vi "SDCP FTOR.vi"(2 "error in (no error)":errorcluster, 3 "FID":u8[](array[numeric])) -> (0 "error out":errorcluster, 1 "Received frames":u8[][](array[numeric]))   [LabVIEW 2020]
uses:
  Typedefs/SDCP - Serial Port Control - Commands.ctl
  Typedefs/SDCP FTOR params.ctl
  <vilib>/Instr/_visa.llb/VISA Flush IO Buffer Mask.ctl
panel:
  out "Timeout errors\nframes":errorcluster[](array[cluster])
  out "timeout\nerrors\nACK":errorcluster[](array[cluster])
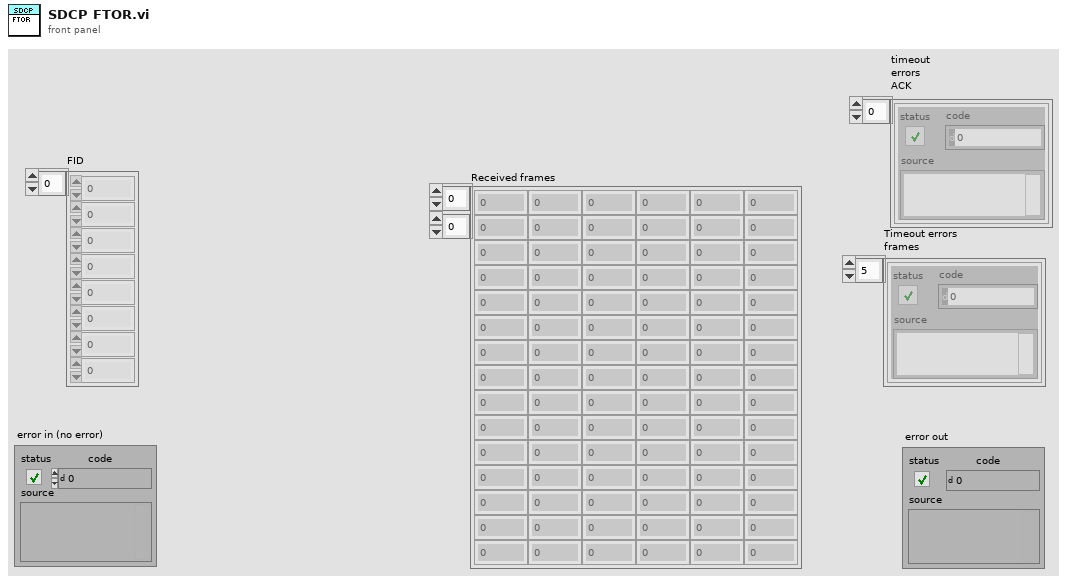
[diagram p1: front panel]
types:
  T1 = typedef "SDCP - Serial Port Control - Commands.ctl" = enum16{"Open", "Read", "Write", "Get instance", "Close"}
  T2 = typedef "SDCP FTOR params.ctl" = cluster{"FID_0":i32, "FID_1":i32, "FID_2":i32, "FID_3":i32, "FID_4":i32, "FID_5":i32, "FID_6":i32, "N_FIDs":i32, "REQ":bool, "ACK":bool}
  T3 = typedef "VISA Flush IO Buffer Mask.ctl" = u16
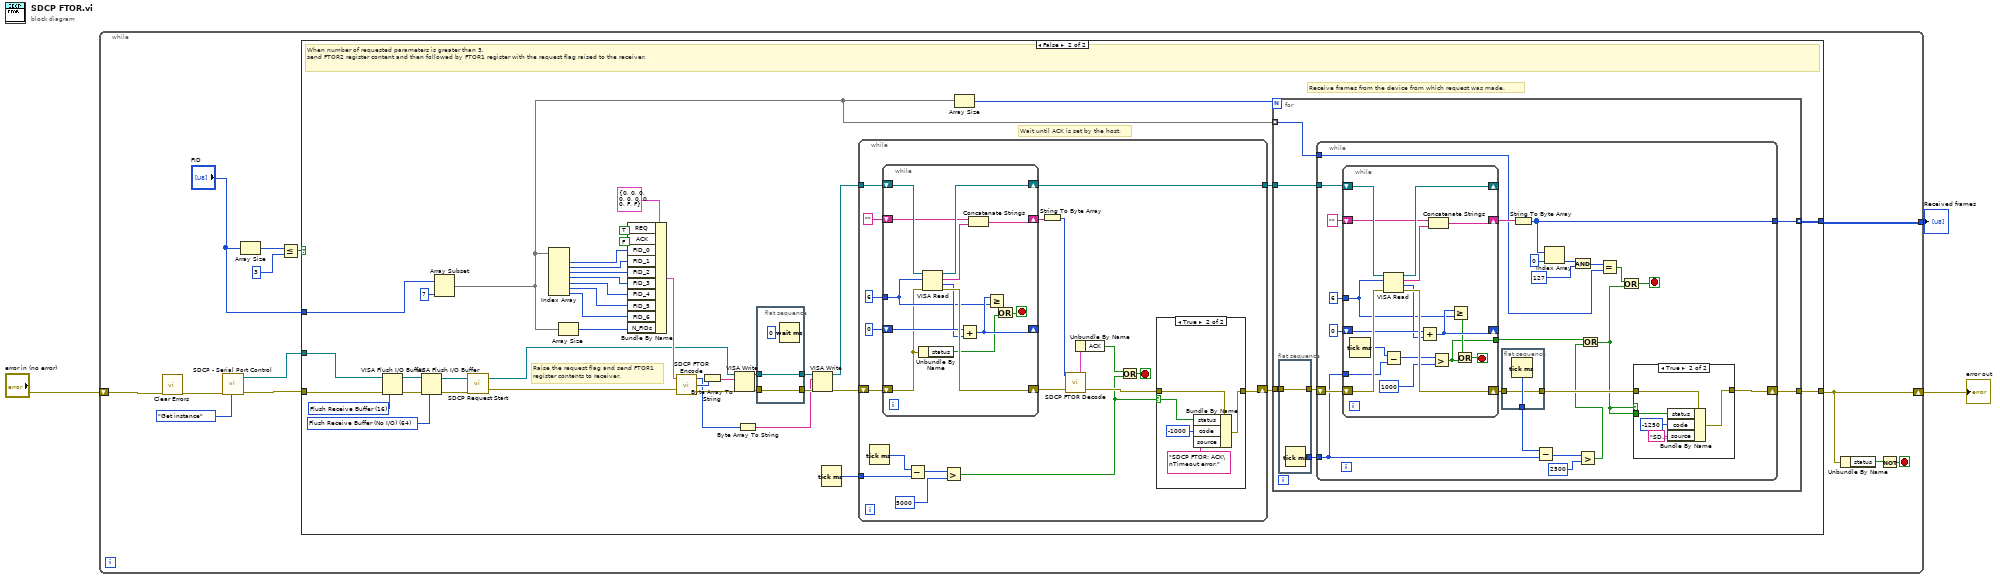
[diagram p0: block diagram]
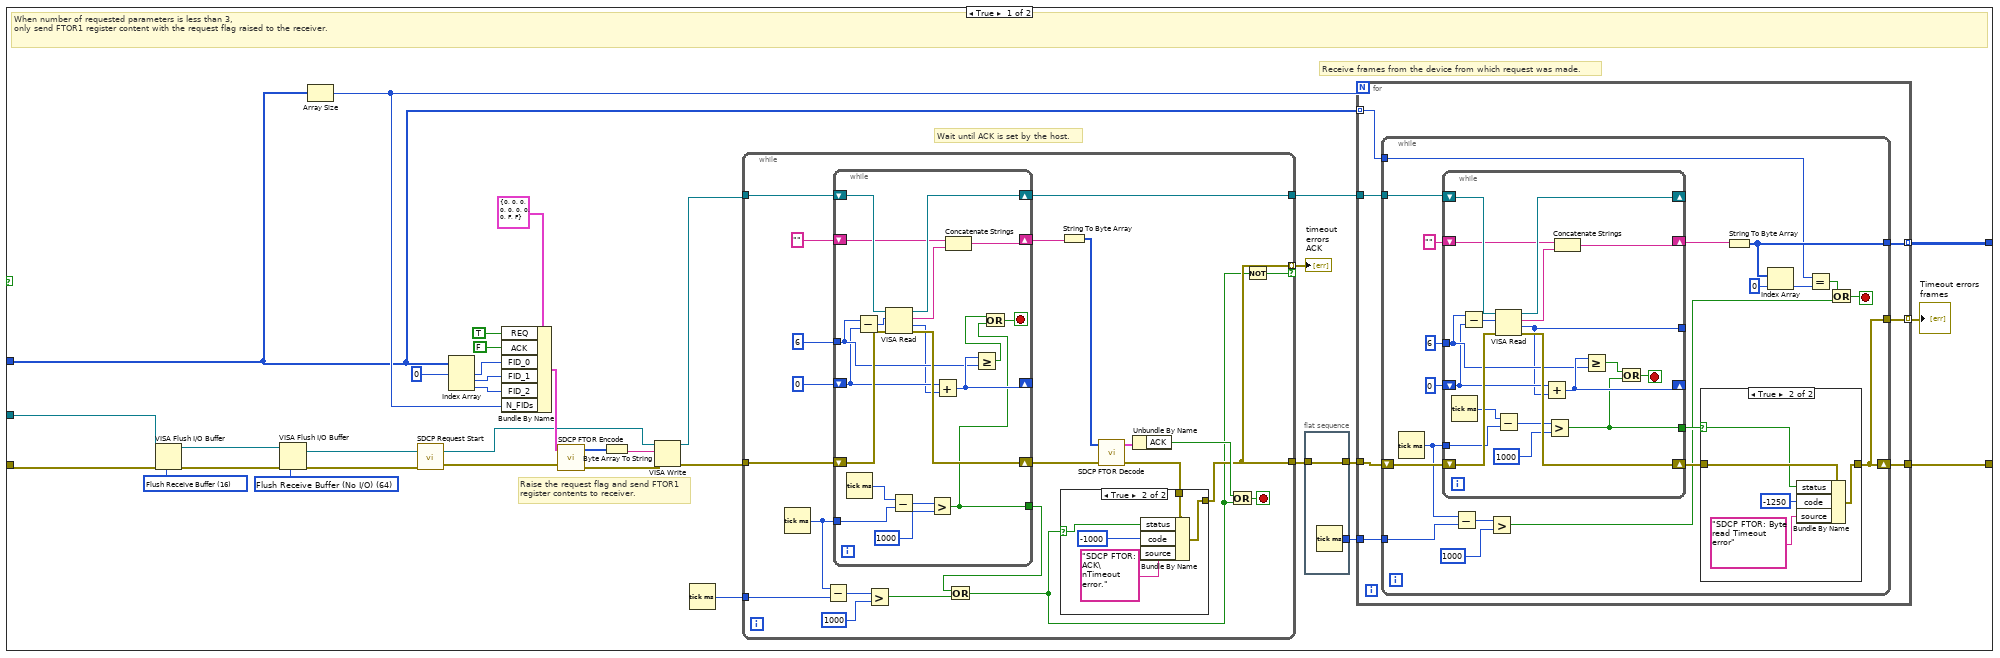
[diagram p2: hidden frame]
diagram:
  n1 = while {
    tunnel: [w9] -> w2
    shift-right: [w6] -> w3
    shift-left: "error in (no error)" -> [w8]
    stop <- w5 stop-if-true
    n2 = call <vilib>:"Clear Errors.vi"("error in (no error)"=w8) -> ("error out"=w7:errorcluster)  [unwired: 5 in, 1 out]
    n3 = call "SDCP - Serial Port Control.vi"("Command"=SDCP_-_Serial_Port_Control_-_Commands."Get instance", "error in (no error)"=w7) -> ("error out"=w12:errorcluster, "VISA out"=w10:refnum<visa-resource-name>)  [unwired: 6 in, 2 out]
    n4 = Array Size(array="FID") -> (size(s)=w15:i32)
    n5 = Less Or Equal?(x=w15, y=3) -> (x <= y?=w13:bool)
    n6 = case shown="False" w13 {
      tunnel: w12 -> [w32 w169]
      tunnel: "FID" -> [w33 w160]
      tunnel: w10 -> [w28 w164]
      tunnel: [w37 w182] -> w9
      tunnel: [w36 w181] -> w6
      frame True {
        w30 = T3 64 items=["Flush Receive Buffer"=16, "Write Transmit Buffer to Device"=32, "Flush Receive Buffer (No I/O)"=64, "Flush Transmit Buffer"=128] ("Mask")
        w31 = T3 16 items=["Flush Receive Buffer"=16, "Write Transmit Buffer to Device"=32, "Flush Receive Buffer (No I/O)"=64, "Flush Transmit Buffer"=128] ("Mask")
        # "Receive frames from the device from which request was made."
        # "Wait until ACK is set by the host."
        # "Raise the request flag and send FTOR1\nregister contents to receiver."
        # "When number of requested parameters is less than 3,\nonly send FTOR1 register content with the request flag raised to the receiver."
        n7 = VISA Flush I/O Buffer(VISA resource name=w28, mask (16)=w31, error in (no error)=w32) -> (VISA resource name out=w27:refnum<visa-resource-name>, error out=w29:errorcluster)
        n8 = VISA Flush I/O Buffer(VISA resource name=w27, mask (16)=w30, error in (no error)=w29) -> (VISA resource name out=w20:refnum<visa-resource-name>, error out=w19:errorcluster)
        n9 = Array Size(array=w33) -> (size(s)=w35:i32)
        n10 = call "SDCP Request Start.vi"("error in (no error)"=w19, "COM Port"=w20) -> ("error out"=w17:errorcluster, "COM Port Out"=w18:refnum<visa-resource-name>)
        n11 = Index Array(array=w33, index #1=0 ("index")) -> (element #1=w46:u8, element #2=w45:u8, element #3=w44:u8)  [unwired: 2 in]
        n12 = Bundle By Name(cluster=T2 {"FID_0"=0, "FID_1"=0, "FID_2"=0, "FID_3"=0, "FID_4"=0, "FID_5"=0, "FID_6"=0, "N_FIDs"=0, "REQ"=FALSE, "ACK"=FALSE}, "REQ"=TRUE, "ACK"=FALSE, "FID_0"=w46, "FID_1"=w45, "FID_2"=w44, "N_FIDs"=w35) -> (w48:T2)
        n13 = call "SDCP FTOR Encode.vi"("error in (no error)"=w17, 5:w48) -> ("error out"=w43:errorcluster, "FTOR1 frame"=w42:u8[])  [unwired: 1 in, 1 out]
        n14 = Byte Array To String(unsigned byte array=w42) -> (string=w41:string)
        n15 = VISA Write(VISA resource name=w18, write buffer=w41, error in (no error)=w43) -> (VISA resource name out=w39:refnum<visa-resource-name>, error out=w40:errorcluster)  [unwired: 1 out]
        n16 = Tick Count (ms)() -> (millisecond timer value=w26:u32)
        n17 = while {
          tunnel: w40 -> [w123]
          tunnel: [w107] -> w23
          tunnel: w39 -> [w118]
          tunnel: [w117] -> w38
          tunnel: w26 -> [w112]
          tunnel: [w107] -> w25 mode=indexing if=w105
          stop <- w116 stop-if-true
          n18 = Tick Count (ms)() -> (millisecond timer value=w113:u32)
          n19 = Subtract(x=w113, y=w112) -> (x-y=w111:u32)
          n20 = while {
            shift-right: [w150] -> w121
            shift-left: w123 -> [w151]
            tunnel: u32 6 ("Read byte count") -> [w135]
            shift-right: [w144] -> _
            shift-left: u32 0 -> [w134]
            shift-right: [w148] -> w117
            shift-left: w118 -> [w149]
            shift-right: [w145] -> w122
            shift-left: "" -> [w147]
            tunnel: w113 -> [w142]
            tunnel: [w137] -> w108
            stop <- w139 stop-if-true
            n21 = Tick Count (ms)() -> (millisecond timer value=w143:u32)
            n22 = Subtract(x=w135, y=w134) -> (x-y=w136:u32)
            n23 = VISA Read(VISA resource name=w149, byte count=w136, error in (no error)=w151) -> (VISA resource name out=w148:refnum<visa-resource-name>, read buffer=w146:string, return count=w133:u32, error out=w150:errorcluster)
            n24 = Subtract(x=w143, y=w142) -> (x-y=w141:u32)
            n25 = Greater?(x=w141, y=u32 1000) -> (0:w137:bool)
            n26 = Add(x=w134, y=w133) -> (x+y=w144:u32)
            n27 = Concatenate Strings(w147, w146) -> (w145:string)
            n28 = Greater Or Equal?(x=w144, y=w135) -> (x >= y?=w138:bool)
            n29 = Or(x=w138, y=w137) -> (x .or. y?=w139:bool)
          }
          n30 = Greater?(x=w111, y=u32 1000) -> (0:w109:bool)
          n31 = Or(x=w108, y=w109) -> (x .or. y?=w106:bool)
          n32 = String To Byte Array(string=w122) -> (unsigned byte array=w120:u8[])
          n33 = call "SDCP FTOR Decode.vi"("error in (no error)"=w121, "FTOR1 frame"=w120) -> ("error out"=w114:errorcluster, "out"=w119:T2)  [unwired: 2 in]
          n34 = case shown="True" w106 {
            selector: w106 -> [_ w128]
            tunnel: w114 -> [w127 w132]
            tunnel: [w127 w131] -> w107
            frame False {
            }
            frame True {
              n35 = Bundle By Name(cluster=w132, "status"=w128, "code"=-1000, "source"="SDCP FTOR: ACK\nTimeout error.") -> (w131:errorcluster)
            }
          }
          n36 = Unbundle By Name(w119) -> ("ACK"=w115:bool)
          n37 = Or(x=w115, y=w106) -> (x .or. y?=w116:bool)
          n38 = Not(x=w106) -> (.not. x?=w105:bool)
        }
        "timeout\nerrors\nACK" <- w25
        n39 = flat-sequence {
          tunnel: [w52] -> w24
          tunnel: w23 -> [w51]
          tunnel: [w51] -> w22
          frame #0 {
            n40 = Tick Count (ms)() -> (millisecond timer value=w52:u32)
          }
        }
        n41 = for {
          N: w35 -> [_]
          tunnel: w22 -> [w59]
          tunnel: w38 -> [w58]
          tunnel: [w57] -> w36
          tunnel: [w56] -> w37 mode=indexing
          tunnel: w33 -> [w55] mode=indexing
          tunnel: w24 -> [w54]
          tunnel: [w53] -> w21 mode=indexing
          n42 = while {
            tunnel: w58 -> [w75]
            tunnel: [w73] -> w56
            shift-right: [w67] -> w57
            shift-left: w59 -> [w79]
            tunnel: w55 -> [w70]
            tunnel: w54 -> [w65]
            tunnel: [w67] -> w53
            stop <- w61 stop-if-true
            n43 = Tick Count (ms)() -> (millisecond timer value=w66:u32)
            n44 = while {
              shift-right: [w103] -> w68
              shift-left: w79 -> [w104]
              tunnel: u32 6 ("Read byte count") -> [w88]
              shift-right: [w97] -> _
              shift-left: u32 0 -> [w87]
              shift-right: [w101] -> _
              shift-left: w75 -> [w102]
              shift-right: [w98] -> w74
              shift-left: "" -> [w100]
              tunnel: w66 -> [w95]
              tunnel: [w90] -> w69
              tunnel: [w86] -> _
              stop <- w92 stop-if-true
              n45 = Tick Count (ms)() -> (millisecond timer value=w96:u32)
              n46 = Subtract(x=w88, y=w87) -> (x-y=w89:u32)
              n47 = VISA Read(VISA resource name=w102, byte count=w89, error in (no error)=w104) -> (VISA resource name out=w101:refnum<visa-resource-name>, read buffer=w99:string, return count=w86:u32, error out=w103:errorcluster)
              n48 = Subtract(x=w96, y=w95) -> (x-y=w94:u32)
              n49 = Add(x=w87, y=w86) -> (x+y=w97:u32)
              n50 = Greater?(x=w94, y=u32 1000) -> (0:w90:bool)
              n51 = Concatenate Strings(w100, w99) -> (w98:string)
              n52 = Greater Or Equal?(x=w97, y=w88) -> (x >= y?=w91:bool)
              n53 = Or(x=w91, y=w90) -> (x .or. y?=w92:bool)
            }
            n54 = Subtract(x=w66, y=w65) -> (x-y=w64:u32)
            n55 = Greater?(x=w64, y=u32 1000) -> (0:w60:bool)
            n56 = case shown="True" w69 {
              selector: w69 -> [_ w83]
              tunnel: w68 -> [w80 w85]
              tunnel: [w80 w84] -> w67
              frame False {
              }
              frame True {
                n57 = Bundle By Name(cluster=w85, "status"=w83, "code"=-1250, "source"="SDCP FTOR: Byte read Timeout error") -> (w84:errorcluster)
              }
            }
            n58 = String To Byte Array(string=w74) -> (unsigned byte array=w73:u8[])
            n59 = Index Array(array=w73, index=0) -> (element=w71:u8)
            n60 = Equal?(x=w70, y=w71) -> (x = y?=w62:bool)
            n61 = Or(x=w62, y=w60) -> (x .or. y?=w61:bool)
          }
        }
        "Timeout errors\nframes" <- w21
      }
      frame False {
        w165 = T3 64 items=["Flush Receive Buffer"=16, "Write Transmit Buffer to Device"=32, "Flush Receive Buffer (No I/O)"=64, "Flush Transmit Buffer"=128] ("Mask")
        w168 = T3 16 items=["Flush Receive Buffer"=16, "Write Transmit Buffer to Device"=32, "Flush Receive Buffer (No I/O)"=64, "Flush Transmit Buffer"=128] ("Mask")
        # "Receive frames from the device from which request was made."
        # "Wait until ACK is set by the host."
        # "Raise the request flag and send FTOR1\nregister contents to receiver."
        # "When number of requested parameters is greater than 3,\nsend FTOR2 register content and then followed by FTOR1 register with the request flag raised to the receiver."
        n62 = VISA Flush I/O Buffer(VISA resource name=w164, mask (16)=w168, error in (no error)=w169) -> (VISA resource name out=w166:refnum<visa-resource-name>, error out=w167:errorcluster)
        n63 = VISA Flush I/O Buffer(VISA resource name=w166, mask (16)=w165, error in (no error)=w167) -> (VISA resource name out=w155:refnum<visa-resource-name>, error out=w154:errorcluster)
        n64 = Array Subset(array=w160, length=7) -> (w158:u8[])  [unwired: 1 in]
        n65 = call "SDCP Request Start.vi"("error in (no error)"=w154, "COM Port"=w155) -> ("error out"=w152:errorcluster, "COM Port Out"=w153:refnum<visa-resource-name>)
        n66 = Index Array(array=w158) -> (element #1=w189:u8, element #2=w188:u8, element #3=w187:u8, element #4=w180:u8, element #5=w179:u8, element #6=w178:u8, element #7=w177:u8)  [unwired: 7 in]
        n67 = Array Size(array=w158) -> (size(s)=w161:i32)
        n68 = Bundle By Name(cluster=T2 {"FID_0"=0, "FID_1"=0, "FID_2"=0, "FID_3"=0, "FID_4"=0, "FID_5"=0, "FID_6"=0, "N_FIDs"=0, "REQ"=FALSE, "ACK"=FALSE}, "REQ"=TRUE, "ACK"=FALSE, "FID_0"=w189, "FID_1"=w188, "FID_2"=w187, "FID_3"=w180, "FID_4"=w179, "FID_5"=w178, "FID_6"=w177, "N_FIDs"=w161) -> (w191:T2)
        n69 = call "SDCP FTOR Encode.vi"("error in (no error)"=w152, 5:w191) -> ("error out"=w186:errorcluster, "FTOR2 frame"=w163:u8[], "FTOR1 frame"=w162:u8[])  [unwired: 1 in]
        n70 = Byte Array To String(unsigned byte array=w163) -> (string=w185:string)
        n71 = VISA Write(VISA resource name=w153, write buffer=w185, error in (no error)=w186) -> (VISA resource name out=w173:refnum<visa-resource-name>, error out=w175:errorcluster)  [unwired: 1 out]
        n72 = Byte Array To String(unsigned byte array=w162) -> (string=w171:string)
        n73 = flat-sequence {
          tunnel: w175 -> [w196]
          tunnel: [w196] -> w174
          tunnel: w173 -> [w195]
          tunnel: [w195] -> w172
          frame #0 {
            n74 = Wait (ms)(milliseconds to wait=u32 0) -> ()  [unwired: 1 out]
          }
        }
        n75 = VISA Write(VISA resource name=w172, write buffer=w171, error in (no error)=w174) -> (VISA resource name out=w170:refnum<visa-resource-name>, error out=w176:errorcluster)  [unwired: 1 out]
        n76 = Tick Count (ms)() -> (millisecond timer value=w157:u32)
        n77 = while {
          tunnel: [w266] -> w183
          tunnel: w170 -> [w265]
          tunnel: w157 -> [w259]
          shift-right: [w256] -> w156
          shift-left: w176 -> [w271]
          stop <- w261 stop-if-true
          n78 = Tick Count (ms)() -> (millisecond timer value=w264:u32)
          n79 = while {
            shift-right: [w294] -> w269
            shift-left: w271 -> [w282]
            tunnel: u32 6 ("Read byte count") -> [w285]
            shift-right: [w286] -> _
            shift-left: u32 0 -> [w291]
            shift-right: [w292] -> w266
            shift-left: w265 -> [w293]
            shift-right: [w287] -> w270
            shift-left: "" -> [w289]
            stop <- w283 stop-if-true
            n80 = Unbundle By Name(w282) -> ("status"=w281:bool)
            n81 = VISA Read(VISA resource name=w293, byte count=w285, error in (no error)=w282) -> (VISA resource name out=w292:refnum<visa-resource-name>, read buffer=w288:string, return count=w290:u32, error out=w294:errorcluster)
            n82 = Add(x=w291, y=w290) -> (x+y=w286:u32)
            n83 = Concatenate Strings(w289, w288) -> (w287:string)
            n84 = Greater Or Equal?(x=w286, y=w285) -> (x >= y?=w284:bool)
            n85 = Or(x=w284, y=w281) -> (x .or. y?=w283:bool)
          }
          n86 = Subtract(x=w264, y=w259) -> (x-y=w263:u32)
          n87 = Greater?(x=w263, y=u32 5000) -> (0:w257:bool)
          n88 = String To Byte Array(string=w270) -> (unsigned byte array=w268:u8[])
          n89 = call "SDCP FTOR Decode.vi"("error in (no error)"=w269, "FTOR1 frame"=w268) -> ("error out"=w258:errorcluster, "out"=w267:T2)  [unwired: 2 in]
          n90 = Unbundle By Name(w267) -> ("ACK"=w260:bool)
          n91 = Or(x=w260, y=w257) -> (x .or. y?=w261:bool)
          n92 = case shown="True" w257 {
            selector: w257 -> [_ w278]
            tunnel: w258 -> [w275 w280]
            tunnel: [w275 w279] -> w256
            frame False {
            }
            frame True {
              n93 = Bundle By Name(cluster=w280, "status"=w278, "code"=-1000, "source"="SDCP FTOR: ACK\nTimeout error.") -> (w279:errorcluster)
            }
          }
        }
        n94 = Array Size(array=w158) -> (size(s)=w184:i32)
        n95 = for {
          N: w184 -> [_]
          tunnel: w156 -> [w198]
          tunnel: w183 -> [w203]
          tunnel: [w202] -> w181
          tunnel: [w201] -> w182 mode=indexing
          tunnel: w158 -> [w200] mode=indexing
          n96 = flat-sequence {
            tunnel: [w205] -> w199
            tunnel: w198 -> [w204]
            tunnel: [w204] -> w197
            frame #0 {
              n97 = Tick Count (ms)() -> (millisecond timer value=w205:u32)
            }
          }
          n98 = while {
            tunnel: w203 -> [w225]
            tunnel: [w223] -> w201
            shift-right: [w210] -> w202
            shift-left: w197 -> [w229]
            tunnel: w200 -> [w218]
            tunnel: w199 -> [w209]
            stop <- w212 stop-if-true
            n99 = while {
              shift-right: [w254] -> w216
              shift-left: w229 -> [w255]
              tunnel: u32 6 ("Read byte count") -> [w245]
              shift-right: [w246] -> _
              shift-left: u32 0 -> [w251]
              shift-right: [w252] -> _
              shift-left: w225 -> [w253]
              shift-right: [w247] -> w224
              shift-left: "" -> [w249]
              tunnel: w209 -> [w243]
              tunnel: [w238] -> w208
              stop <- w239 stop-if-true
              n100 = Tick Count (ms)() -> (millisecond timer value=w244:u32)
              n101 = VISA Read(VISA resource name=w253, byte count=w245, error in (no error)=w255) -> (VISA resource name out=w252:refnum<visa-resource-name>, read buffer=w248:string, return count=w250:u32, error out=w254:errorcluster)
              n102 = Subtract(x=w244, y=w243) -> (x-y=w242:u32)
              n103 = Add(x=w251, y=w250) -> (x+y=w246:u32)
              n104 = Concatenate Strings(w249, w248) -> (w247:string)
              n105 = Greater?(x=w242, y=u32 1000) -> (0:w238:bool)
              n106 = Greater Or Equal?(x=w246, y=w245) -> (x >= y?=w240:bool)
              n107 = Or(x=w240, y=w238) -> (x .or. y?=w239:bool)
            }
            n108 = flat-sequence {
              tunnel: [w237] -> w217
              tunnel: w216 -> [w236]
              tunnel: [w236] -> w211
              frame #0 {
                n109 = Tick Count (ms)() -> (millisecond timer value=w237:u32)
              }
            }
            n110 = String To Byte Array(string=w224) -> (unsigned byte array=w223:u8[])
            n111 = Subtract(x=w217, y=w209) -> (x-y=w215:u32)
            n112 = Index Array(array=w223, index=0) -> (element=w221:u8)
            n113 = And(x=w221, y=u8 127) -> (x .and. y?=w219:u8)
            n114 = Greater?(x=w215, y=u32 2500) -> (0:w207:bool)
            n115 = Or(x=w208, y=w207) -> (x .or. y?=w206:bool)
            n116 = Equal?(x=w219, y=w218) -> (x = y?=w213:bool)
            n117 = Or(x=w213, y=w206) -> (x .or. y?=w212:bool)
            n118 = case shown="True" w206 {
              tunnel: w211 -> [w230 w235]
              tunnel: [w230 w234] -> w210
              tunnel: w206 -> [_ w233]
              frame False {
              }
              frame True {
                n119 = Bundle By Name(cluster=w235, "status"=w233, "code"=-1250, "source"="SDCP FTOR: Byte read Timeout error") -> (w234:errorcluster)
              }
            }
          }
        }
      }
    }
    n120 = Unbundle By Name(w6) -> ("status"=w4:bool)
    n121 = Not(x=w4) -> (.not. x?=w5:bool)
  }
  "error out" <- w3
  "Received frames" <- w2
